vi "BallandBeam(NoLPF).vi"() -> ()   [LabVIEW 2017]
uses:
  <vilib>/Platform/TimedLoop/XDataNode/timing_clust.ctl
  <vilib>/Platform/TimedLoop/XDataNode/nitl_modes.ctl
  <vilib>/Platform/TimedLoop/XDataNode/wakeup.ctl
  <vilib>/myRIO/Instrument Drivers/Onboard IO/AI/vis/Read.vi
  <vilib>/myRIO/Instrument Drivers/Onboard IO/AO/vis/Write.vi
  <vilib>/myRIO/Instrument Drivers/Onboard IO/AI/vis/Smart Open.vi
  <vilib>/Utility/error.llb/Error Cluster From Error Code.vi
  <vilib>/myRIO/Common/Instrument Driver Framework/myRIO v1.0/AI/vis/myRIO v1.0 Read AI.vi
  <vilib>/myRIO/Instrument Drivers/Onboard IO/AO/vis/Smart Open.vi
  <vilib>/myRIO/Common/Instrument Driver Framework/myRIO v1.0/AO/vis/myRIO v1.0 Write AO.vi
  <vilib>/platform/TimedLoop/XDataNode/XDataNode.xnode
  <vilib>/Platform/TimedLoop/XDataNode/XDNodeRunTimeDep.lvlib
panel:
  in  "Period":i64
  out "Theta Output 2":dbl
  out "X Error 4":dbl
  out "X Error 3":dbl(graph)=-0.6885397082002527
  in  "Theta Bound 2":dbl=3.0
  in  "Kp 2":dbl=0.5
  in  "Kd 2":dbl
  in  "X disire 2":dbl
  out "Vout 2":dbl
  in  "Vout Bound 2":dbl=4.5
  in  "Kp1 2":dbl=1.0
  out "Theta 2":dbl
  in  "t offset 2":dbl
  in  "t amp 2":dbl
  out "Position 2":dbl
  in  "x offset 2":dbl
  in  "x amp 2":dbl
  out "Theta voltage 2":dbl
  out "X voltage 2":dbl
  in  "stop 2":bool
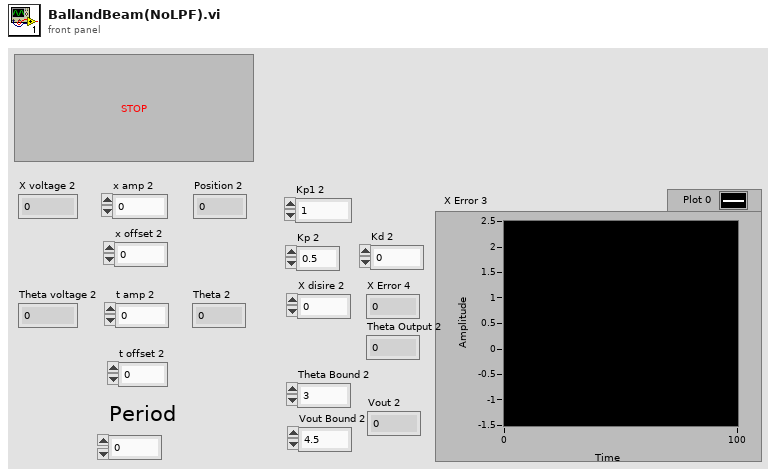
[diagram p1: front panel]
types:
  T1 = typedef "XDNodeRunTimeDep.lvlib/timing_clust.ctl" = cluster{"Expected End [f-1]":u64, "Actual End [f-1]":u64, "Finished Late? [f-1]":bool, "Expected End [i-1]":u64, "Actual End [i-1]":u64, "Finished Late? [i-1]":bool, "Expected Start [i]":u64, "Actual Start [i]":u64, "Expected Start [f]":u64, "Actual Start [f]":u64, "Source Name":string, "Structure Name":string, "Period":i64, "Deadline":i64, "Offset":i64, "Start":i64, "Priority":i32, "Timeout":i32, "Mode":T2, "Wakeup Reason":T3, "Error":errorcluster, "Source Type":string, "Secondary Source Type":string, "Global End Time":u64, "Global Start Time":u64, "Frame Duration":u64, "Iteration Duration":u64, "Assigned CPU":i32, "I/O Scan Engine Mode":u32}
  T2 = typedef "XDNodeRunTimeDep.lvlib/nitl_modes.ctl" = enum32{"No Change", "Process missed periods, maintain original phase", "Discard missed periods, maintain original phase", "Process missed periods, ignore original phase", "Discard missed periods, ignore original phase"}
  T3 = typedef "XDNodeRunTimeDep.lvlib/wakeup.ctl" = enum32{"Normal", "Aborted", "Asynchronous wakeup", "Timing source error", "Timed loop error", "Timeout"}
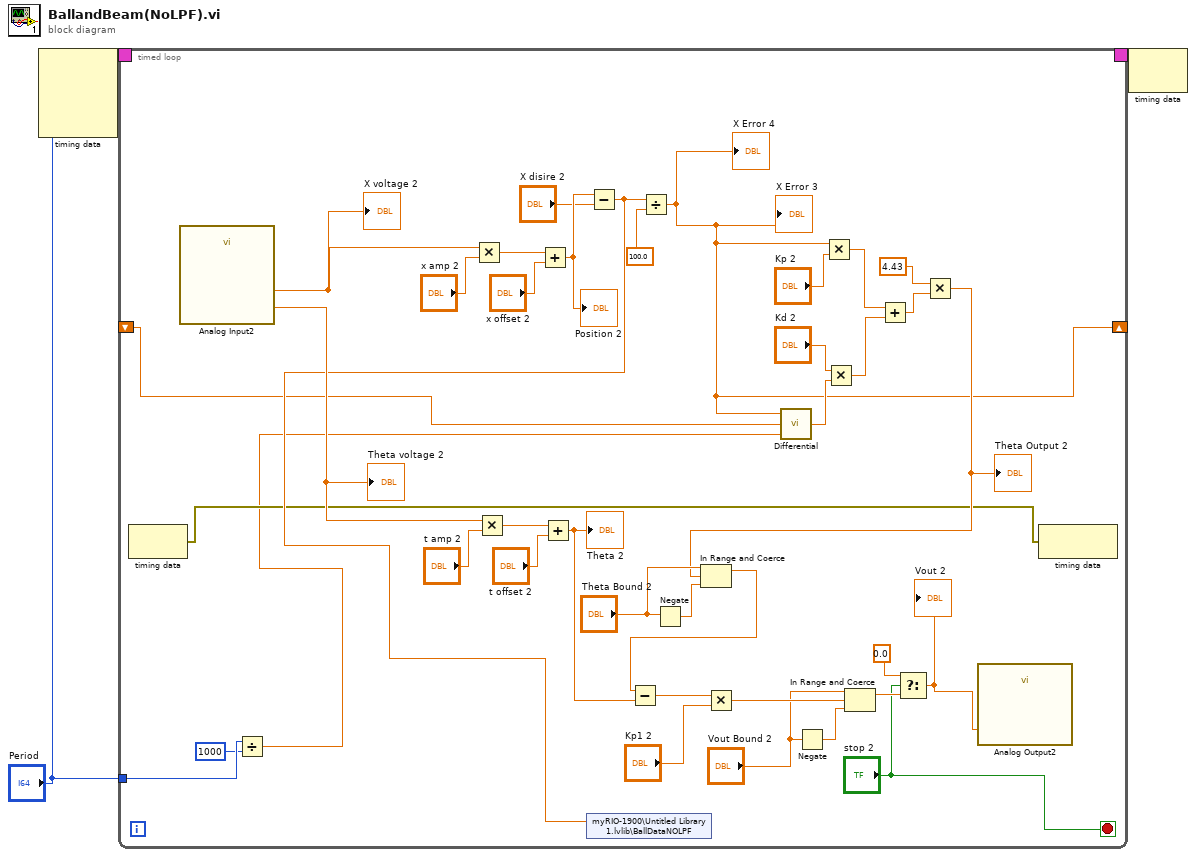
[diagram p0: block diagram]
diagram:
  n1 = node-c288("Period") -> (w3:T1)  [unwired: 3 in]
  n2 = timed-loop {
    timing: w3 -> [_]
    timing-out: [_] -> w2
    shift-right: [w8] -> _
    shift-left: _ -> [w9]
    tunnel: "Period" -> [w6]
    stop <- "stop 2" stop-if-true
    n3 = node-c288() -> (w7:errorcluster)  [unwired: 1 in]
    n4 = call "Analog Input2"() -> ("C/AI0"=w14:dbl, "C/AI1"=w13:dbl)  [unwired: 25 in, 1 out]
    "X voltage 2" <- w14
    "Theta voltage 2" <- w13
    n5 = Divide(x=w6, y=i64 1000) -> (x/y=w4:dbl)
    n6 = Multiply(x=w14, y="x amp 2") -> (x*y=w42:dbl)
    n7 = Multiply(x=w13, y="t amp 2") -> (x*y=w39:dbl)
    n8 = Add(x=w42, y="x offset 2") -> (x+y=w20:dbl)
    "Position 2" <- w20
    n9 = Add(x=w39, y="t offset 2") -> (x+y=w30:dbl)
    "Theta 2" <- w30
    n10 = Subtract(x=w20, y="X disire 2") -> (x-y=w11:dbl)
    n11 = shared-variable "myRIO-1900\\Untitled Library 1.lvlib\\BallDataNOLPF"(w11) -> ()  [unwired: 1 in, 1 out]
    n12 = Divide(x=w11, y=100.0) -> (x/y=w8:dbl)
    "X Error 3" <- w8
    "X Error 4" <- w8
    n13 = Negate(x="Theta Bound 2") -> (-x=w22:dbl)
    n14 = call "Differential.vi"("Ts"=w4, "X[k-1]"=w9, "X[k]"=w8) -> ("dX"=w28:dbl)
    n15 = Negate(x="Vout Bound 2") -> (-x=w34:dbl)
    n16 = Multiply(x=w8, y="Kp 2") -> (x*y=w25:dbl)
    n17 = Multiply(x="Kd 2", y=w28) -> (x*y=w24:dbl)
    n18 = Add(x=w25, y=w24) -> (x+y=w16:dbl)
    n19 = Multiply(x=4.43, y=w16) -> (x*y=w15:dbl)
    "Theta Output 2" <- w15
    n20 = In Range and Coerce(upper limit="Theta Bound 2", x=w15, lower limit=w22) -> (coerced(x)=w21:dbl)  [unwired: 1 out]
    n21 = Subtract(x=w21, y=w30) -> (x-y=w29:dbl)
    n22 = Multiply(x=w29, y="Kp1 2") -> (x*y=w33:dbl)
    n23 = In Range and Coerce(upper limit="Vout Bound 2", x=w33, lower limit=w34) -> (coerced(x)=w32:dbl)  [unwired: 1 out]
    n24 = Select(t=0.0, s="stop 2", f=w32) -> (s? t:f=w12:dbl)
    "Vout 2" <- w12
    n25 = call "Analog Output2"("C/AO0"=w12) -> ()  [unwired: 26 in, 1 out]
    n26 = node-c288(w7) -> ()  [unwired: 1 out]
  }
  n27 = node-c288(w2) -> ()  [unwired: 1 out]
